vi "filters_load_xml.vi"(8 "error in":errorcluster, 10 "child node in":refnum<k20>) -> (0 "error out":errorcluster, 2 "child node out":refnum<k20>, 3 "Filter Settings":T1)   [LabVIEW 2012]
doc: "Loads filter settings from xml. Expected format:\n\n<CounterFilterMinimum>\n<bin>%u\\t</bin>\n</CounterFilterMinimum>\n<ROIFiltersMinimum>\n<shot>%u\\t</shot>\n</ROIFiltersMinimum>\n\nMTL 2012 Dec 31"
uses:
  filters.ctl
  <vilib>/xml/Close Reference(Node).vi
  <resource>/objmgr/DOMUserDefRef.rc
  <vilib>/xml/NI_XML.lvlib
panel:
  # "Regions of Interest -->"
  # "Shots\n   |\n  V"
  # "Counters -->"
  # "Counter\n    bins\n       |\n      V"
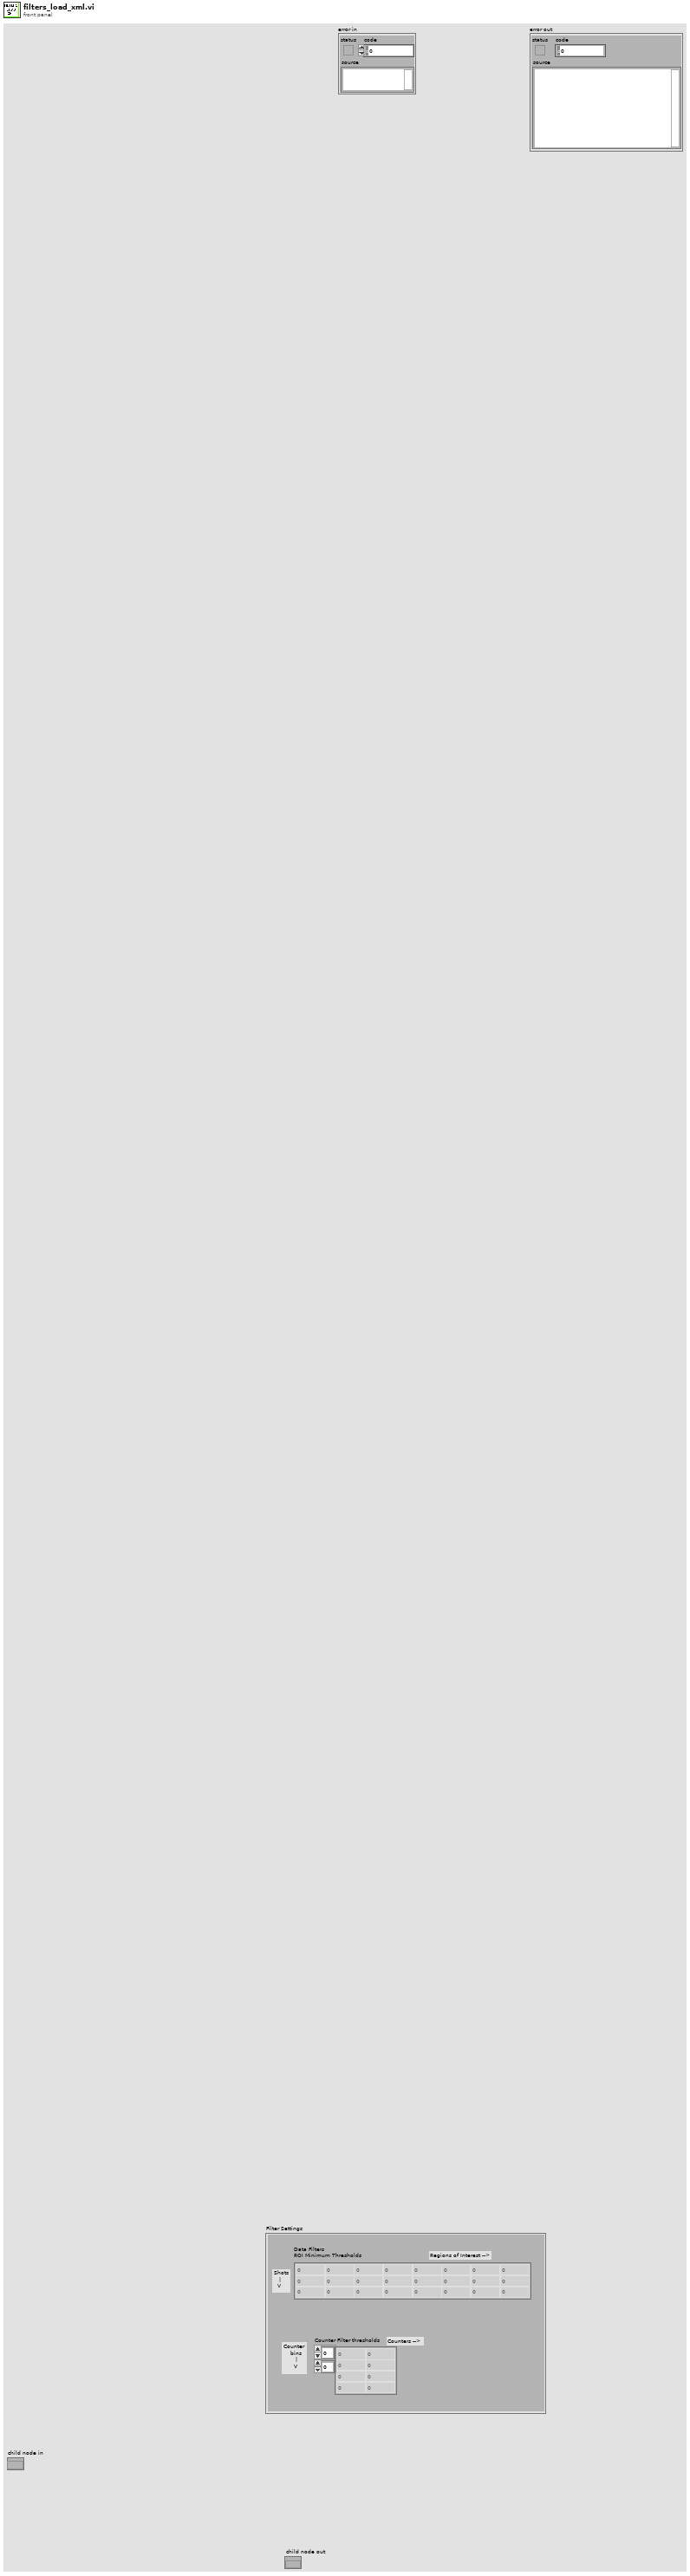
[diagram p1: front panel]
types:
  T1 = typedef "filters.ctl" = cluster{"Counter Filter thresholds":u32[][], "Data Filters\nROI Minimum Thresholds":u64[][]}
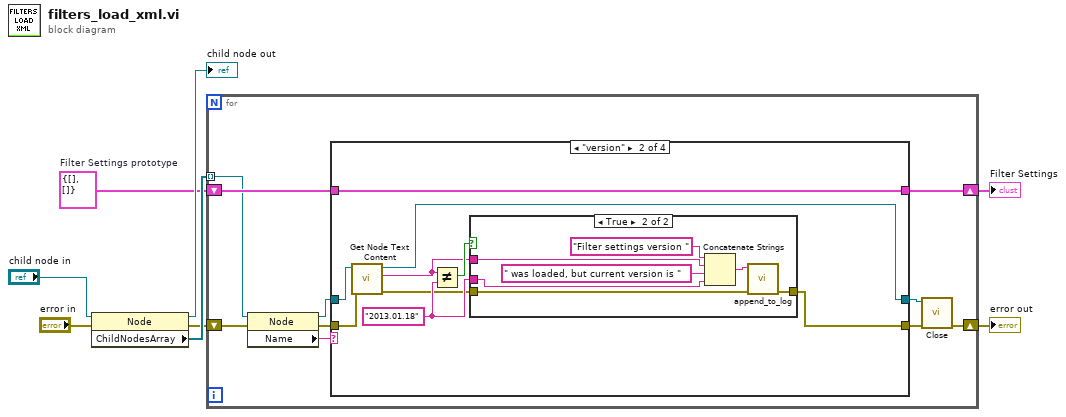
[diagram p0: block diagram]
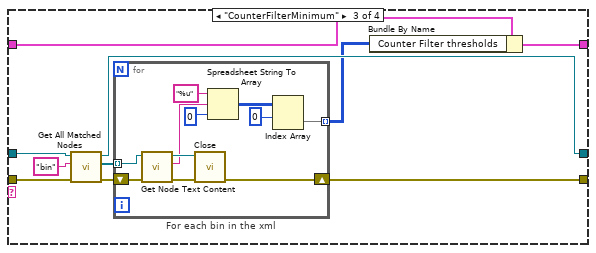
[diagram p4: hidden frame]
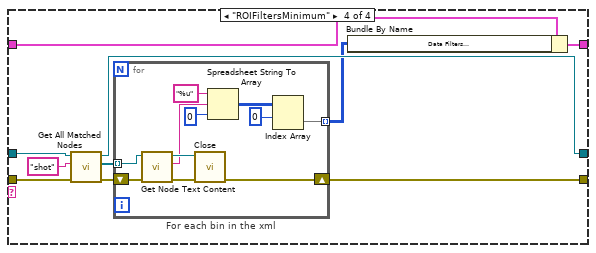
[diagram p5: hidden frame]
diagram:
  w2 = T1 {"Counter Filter thresholds"=[], "Data Filters\nROI Minimum Thresholds"=[]}  # Filter Settings prototype
  n1 = property class="Node"(reference="child node in", error in="error in") -> (reference out=→"child node out":refnum<k20>, error out=w6:errorcluster, "ChildNodesArray"=w8:refnum<k20>[])
  n2 = for {
    tunnel: w8 -> [w9] mode=indexing
    shift-right: [w15] -> w1
    shift-left: w2 -> [w16]
    shift-right: [w12] -> w3
    shift-left: w6 -> [w10]
    n3 = property class="Node"(reference=w9, error in=w10) -> (reference out=w17:refnum<k20>, error out=w13:errorcluster, "Name"=w18:string)
    n4 = case shown="\"version\"" w18 {
      tunnel: w17 -> [w20 w25 w45 w66]
      tunnel: w16 -> [w21 w26 w48 w69]
      tunnel: [w21 w26 w47 w68] -> w15
      tunnel: [w20 w23 w44 w65] -> w14
      tunnel: w13 -> [w19 w24 w43 w64]
      tunnel: [w19 w22 w40 w61] -> w11
      frame "None", Default {
      }
      frame "version" {
        w28 = "2013.01.18" ("y")
        n5 = call <vilib>:"Get Node Text Content.vi"("error in (no error)"=w24, "node in"=w25) -> ("error out"=w27:errorcluster, "node text"=w29:string, "node out"=w23:refnum<k20>)  [unwired: 7 in]
        n6 = Not Equal?(x=w29, y=w28) -> (x != y?=w30:bool)
        n7 = case shown="True" w30 {
          tunnel: w29 -> [_ w37]
          tunnel: w28 -> [_ w35]
          tunnel: w27 -> [w31 w33]
          tunnel: [w31 w32] -> w22
          frame False {
          }
          frame True {
            n8 = Concatenate Strings("Filter settings version " ("string"), w37, " was loaded, but current version is " ("string"), w35) -> (w34:string)
            n9 = call "append_to_log.vi"("error in"=w33, "string"=w34) -> ("error out"=w32:errorcluster)  [unwired: 8 in, 1 out]
          }
        }
      }
      frame "CounterFilterMinimum" {
        n10 = call <vilib>:"Get All Matched Nodes.vi"("error in (no error)"=w43, "XPath expression"="bin", "node in"=w45) -> ("error out"=w41:errorcluster, "node result array"=w46:refnum<k20>[], "node out"=w44:refnum<k20>)  [unwired: 6 in]
        n11 = for "For each bin in the xml" {
          tunnel: w46 -> [w58] mode=indexing
          shift-right: [w59] -> w40
          shift-left: w41 -> [w51]
          tunnel: [w53] -> w39 mode=indexing
          n12 = call <vilib>:"Get Node Text Content.vi"("error in (no error)"=w51, "node in"=w58) -> ("error out"=w50:errorcluster, "node text"=w56:string, "node out"=w57:refnum<k20>)  [unwired: 7 in]
          n13 = call-poly <vilib>:"Close.vi"("error in (no error)"=w50, "node"=w57) -> ("error out"=w59:errorcluster)  [unwired: 7 in]
          n14 = Spreadsheet String To Array(format string="%u", spreadsheet string=w56, array type (2D Dbl)=u32 0 ("dimension size")) -> (array=w55:u32[][])  [unwired: 1 in]
          n15 = Index Array(array=w55, index (row)=0) -> (element=w53:u32[])  [unwired: 1 in]
        }
        n16 = Bundle By Name(cluster=w48, "Counter Filter thresholds"=w39) -> (w47:T1)
      }
      frame "ROIFiltersMinimum" {
        n17 = call <vilib>:"Get All Matched Nodes.vi"("error in (no error)"=w64, "XPath expression"="shot", "node in"=w66) -> ("error out"=w62:errorcluster, "node result array"=w67:refnum<k20>[], "node out"=w65:refnum<k20>)  [unwired: 6 in]
        n18 = for "For each bin in the xml" {
          tunnel: w67 -> [w79] mode=indexing
          shift-right: [w80] -> w61
          shift-left: w62 -> [w72]
          tunnel: [w74] -> w60 mode=indexing
          n19 = call <vilib>:"Get Node Text Content.vi"("error in (no error)"=w72, "node in"=w79) -> ("error out"=w71:errorcluster, "node text"=w77:string, "node out"=w78:refnum<k20>)  [unwired: 7 in]
          n20 = call-poly <vilib>:"Close.vi"("error in (no error)"=w71, "node"=w78) -> ("error out"=w80:errorcluster)  [unwired: 7 in]
          n21 = Spreadsheet String To Array(format string="%u", spreadsheet string=w77, array type (2D Dbl)=u64 0 ("dimension size")) -> (array=w76:u64[][])  [unwired: 1 in]
          n22 = Index Array(array=w76, index (row)=0) -> (element=w74:u64[])  [unwired: 1 in]
        }
        n23 = Bundle By Name(cluster=w69, "Data Filters\nROI Minimum Thresholds"=w60) -> (w68:T1)
      }
    }
    n24 = call-poly <vilib>:"Close.vi"("error in (no error)"=w11, "node"=w14) -> ("error out"=w12:errorcluster)  [unwired: 7 in]
  }
  "error out" <- w3
  "Filter Settings" <- w1
